vi "Delete Int16Array DVR.vi"(8 "error in (no error)":errorcluster, 11 "Int16Array DVR in":refnum<data-value>) -> (0 "error out":errorcluster, 3 "Int16Array out":refnum<class "Int16Array.lvclass">)   [LabVIEW 2013, in "MDSplus.lvlib" / "Int16Array.lvclass"]
uses:
  <vilib>/MDSplus/Classes/Data_Class/Array_Class/Int16Array_Class/Int16Array.lvclass
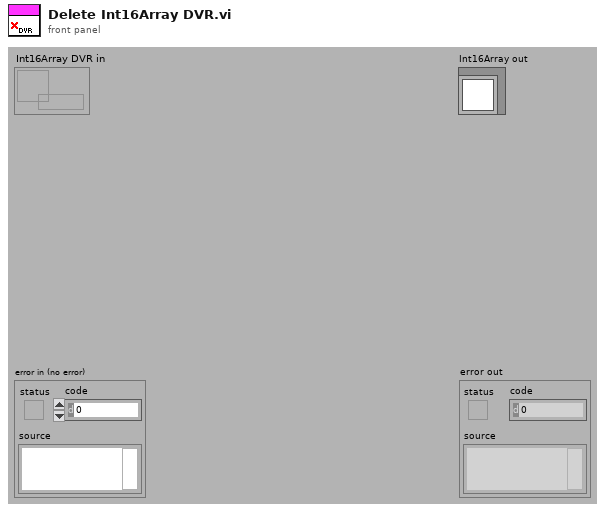
[diagram p1: front panel]
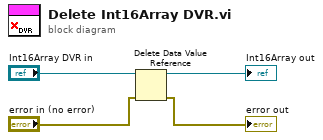
[diagram p0: block diagram]
diagram:
  n1 = Delete Data Value Reference(data value reference="Int16Array DVR in", error in="error in (no error)") -> (data value=→"Int16Array out":refnum<class "Int16Array.lvclass">, error out=→"error out":errorcluster)
